vi "Scan Setup.vi"(8 "error in (no error)":errorcluster, 11 "Double Scanner in":refnum<class "Double Scanner.lvclass">) -> (0 "error out":errorcluster, 3 "Double Scanner out":refnum<class "Double Scanner.lvclass">)   [LabVIEW 2012, in "Double Scanner.lvclass"]
doc: "Configure the Instrument based on the class member fields. This step comes after the user has closed the \"Scan Setup\" window and before the actual scan -- so instruments are configured with the user's specified settings."
uses:
  Double Scanner.lvclass
  Double Scanner.lvclass/Double Scanner.ctl
  Scanner/Scanner.lvclass
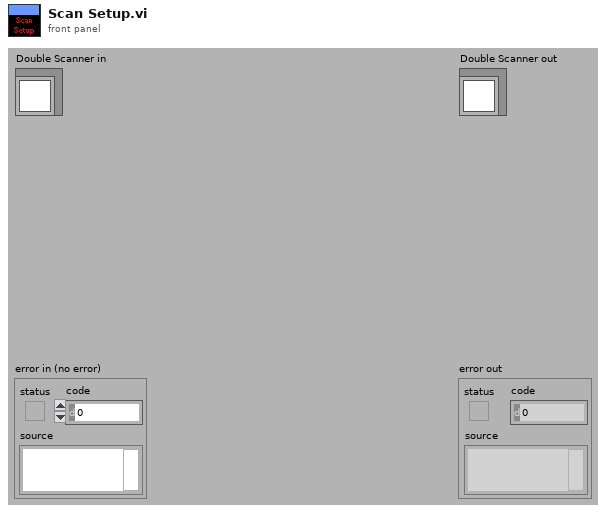
[diagram p1: front panel]
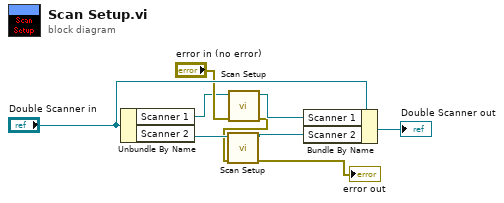
[diagram p0: block diagram]
diagram:
  n1 = Unbundle By Name("Double Scanner in") -> ("Scanner 1"=w5:refnum<class "Scanner.lvclass">, "Scanner 2"=w3:refnum<class "Scanner.lvclass">)
  n2 = call-dynamic "Scan Setup.vi"("error in (no error)"="error in (no error)", "Scanner in"=w5) -> ("error out"=w2:errorcluster, "Scanner out"=w7:refnum<class "Scanner.lvclass">)  [unwired: 8 in]
  n3 = call-dynamic "Scan Setup.vi"("error in (no error)"=w2, "Scanner in"=w3) -> ("error out"=→"error out":errorcluster, "Scanner out"=w4:refnum<class "Scanner.lvclass">)  [unwired: 8 in]
  n4 = Bundle By Name(cluster="Double Scanner in", "Scanner 1"=w7, "Scanner 2"=w4) -> (→"Double Scanner out":refnum<class "Double Scanner.lvclass">)
